vi "Make Encoder JSON.vi"(9 "Force":bool, 10 "Encoder prev":T1={"type"="Encoder", "device"="", "name"="", "data"={"<init"=FALSE, ">count"=0.0, ">period"=0.0, "<samples_to_avg"=0, "<offset"=0.0, "<channel_a"=0, "<channel_b"=0}}, 11 "Encoder new":T1={"type"="Encoder", "device"="", "name"="", "data"={"<init"=FALSE, ">count"=0.0, ">period"=0.0, "<samples_to_avg"=0, "<offset"=0.0, "<channel_a"=0, "<channel_b"=0}}) -> (3 "delta JSON":string)   [LabVIEW 2019]
uses:
  Encoder data protoo.ctl
  Encoder proto.ctl
panel:
  out "Complete JSON":string
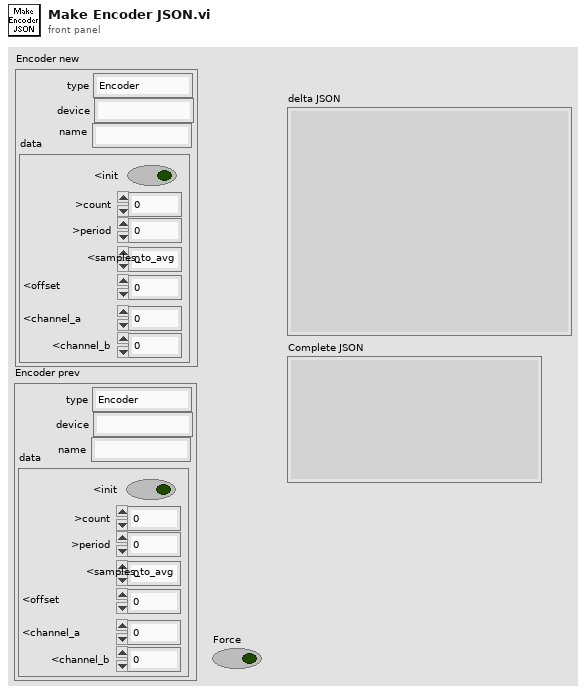
[diagram p1: front panel]
types:
  T1 = typedef "Encoder proto.ctl" = cluster{"type":string, "device":string, "name":string, "data":T2}
  T2 = typedef "Encoder data protoo.ctl" = cluster{"<init":bool, ">count":dbl, ">period":dbl, "<samples_to_avg":i32, "<offset":dbl, "<channel_a":i32, "<channel_b":i32}
  T3 = cluster{"type":bool, "device":bool, "name":bool, "data":cluster{"<init":bool, ">count":bool, ">period":bool, "<samples_to_avg":bool, "<offset":bool, "<channel_a":bool, "<channel_b":bool}}
  T4 = cluster{"<init":bool, ">count":bool, ">period":bool, "<samples_to_avg":bool, "<offset":bool, "<channel_a":bool, "<channel_b":bool}
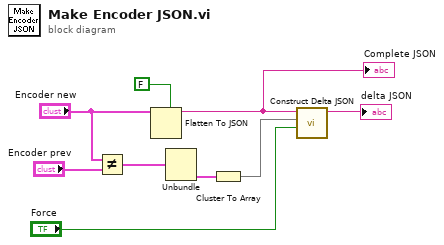
[diagram p0: block diagram]
diagram:
  n1 = Not Equal?(x="Encoder new", y="Encoder prev") -> (x != y?=w2:T3)
  n2 = Flatten To JSON(enable LabVIEW extensions? (T)=FALSE, anything="Encoder new") -> (JSON string=w1:string)  [unwired: 1 in, 1 out]
  "Complete JSON" <- w1
  n3 = Unbundle(w2) -> ("data"=w6:T4)  [unwired: 3 out]
  n4 = Cluster To Array(cluster=w6) -> (array=w4:bool[])
  n5 = call "Construct Delta JSON.vi"("Force"="Force", "Checked Items"=w4, "JSON string"=w1) -> ("Delta JSON"=→"delta JSON":string)  [unwired: 8 in]
